vi "GraphAttribute.vi"() -> ()   [LabVIEW 2012]
panel:
  in  "布尔 3":bool
  in  "布尔 2":bool
  in  "布尔":bool
  in  "选项卡控件":enum32{"曲线", "文本", "信息"}(tab)
  in  "曲线":i32(listbox)
  in  "颜色盒 6":u32(colorbox) caption="颜色"
  in  "下拉列表 13":u16(ring) caption="线条宽度" items=["0", "1", "2", "3", "4", "5"]
  in  "下拉列表 2":u16(ring) caption="线条样式" items=["实线", "粗虚线", "细虚线", "点划线", "双点划线"]
  in  "下拉列表 4":u16(ring) caption="直方图"
  in  "下拉列表 5":u16(ring) caption="插值"
  in  "颜色盒 4":u32(colorbox) caption="点样式"
  in  "填充基线":u16(ring) items=["无", "零", "负无穷大", "正无穷大"]
  in  "加粗":bool
  in  "大小":u16(ring)
  in  "文本":string
  in  "文本":i32(listbox)
  in  "字体":u16(ring)
  in  "颜色":u16(ring)
  in  "斜体":bool
  in  "下划线":bool
  in  "格式":u16(ring) items=["十进制", "科学值"]
  in  "图例 9":bool
  in  "图例 2":bool
  in  "图例":bool
  in  "图例 3":bool
  in  "图例 4":bool
  in  "图例 5":bool
  in  "图例 6":bool
  in  "图例 7":bool
  in  "图例 8":bool
  in  "光标列表":u16(ring) items=["单光标", "双光标", "峰值光标"]
  in  "数量":dbl
  in  "排列":u16(ring) items=["幅值"]
  in  "精度":dbl=3.0
  # "光标"
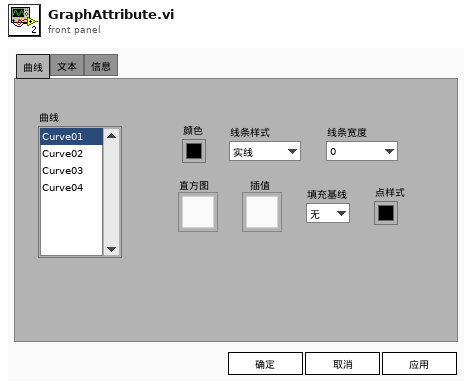
[diagram p1: front panel]
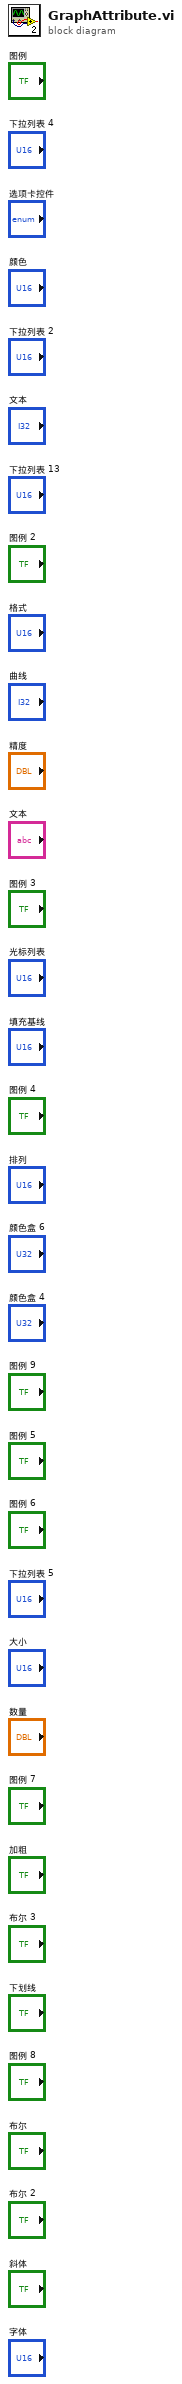
[diagram p0: block diagram]
diagram:
